vi "Save_SpectralGateSweep.vi"(0 "Refnum in":refnum<k34>, 1 "Integrated Emission":dbl[](array[numeric]), 2 "Capture number":i32, 7 "Image":dbl[][](array[numeric]), 11 "error in (no error)":errorcluster, 12 "Gate Delay array":dbl[](array[numeric]), 13 "Wavelength Array":dbl[](array[numeric])) -> (4 "Refnum out":refnum<k34>, 15 "error out":errorcluster)   [LabVIEW 2017]
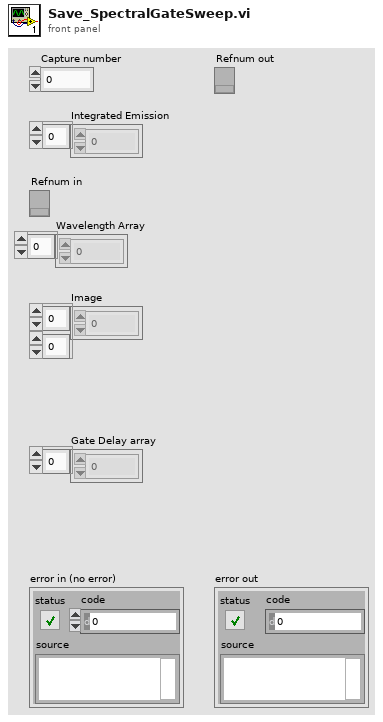
[diagram p1: front panel]
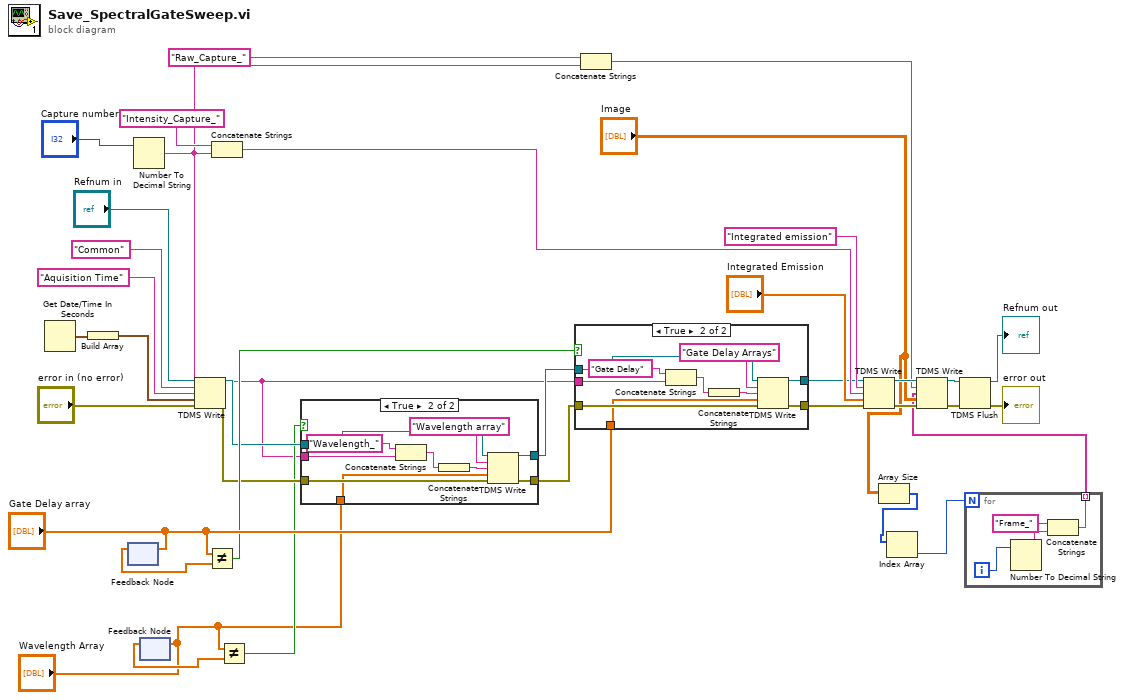
[diagram p0: block diagram]
diagram:
  n1 = Get Date/Time In Seconds() -> (seconds since 1Jan1904=w14:timestamp)
  n2 = Build Array(w14) -> (w19:timestamp[])
  n3 = feedback #1() -> (w17:dbl[])  [unwired: 1 in]
  n4 = feedback-in #1("Gate Delay array") -> ()
  n5 = Number To Decimal String(number="Capture number") -> (decimal integer string=w1:string)  [unwired: 1 in]
  n6 = feedback #2() -> (w4:dbl[])  [unwired: 1 in]
  n7 = feedback-in #2("Wavelength Array") -> ()
  n8 = TDMS Write(0:"Refnum in", 5:"Common" ("group name in (Untitled)"), 7:"Aquisition Time", 9:w19, 11:"error in (no error)") -> (4:w8:refnum<k34>, 15:w7:errorcluster)  [unwired: 1 in, 2 out]
  n9 = Not Equal?(x="Gate Delay array", y=w17) -> (x != y?=w15:bool)
  n10 = Concatenate Strings("Intensity_Capture_" ("group name in (Untitled)"), w1) -> (w24:string)
  n11 = Not Equal?(x="Wavelength Array", y=w4) -> (x != y?=w3:bool)
  n12 = case shown="True" w3 {
    tunnel: w8 -> [w38 w48]
    tunnel: w7 -> [w37 w47]
    tunnel: [w38 w46] -> w6
    tunnel: [w37 w45] -> w5
    tunnel: "Wavelength Array" -> [_ w42]
    tunnel: w1 -> [_ w39]
    frame False {
    }
    frame True {
      n13 = Concatenate Strings("Wavelength_" ("string"), w39) -> (w41:string)
      n14 = Concatenate Strings(w41) -> (w43:string)
      n15 = TDMS Write(0:w48, 5:"Wavelength array" ("group name in (Untitled)"), 7:w43, 9:w42, 11:w47) -> (4:w46:refnum<k34>, 15:w45:errorcluster)  [unwired: 1 in, 2 out]
    }
  }
  n16 = case shown="True" w15 {
    tunnel: w6 -> [w50 w60]
    tunnel: w5 -> [w49 w59]
    tunnel: [w50 w58] -> w21
    tunnel: [w49 w57] -> w22
    tunnel: "Gate Delay array" -> [_ w54]
    tunnel: w1 -> [_ w51]
    frame False {
    }
    frame True {
      n17 = Concatenate Strings("Gate Delay" ("string"), w51) -> (w53:string)
      n18 = Concatenate Strings(w53) -> (w55:string)
      n19 = TDMS Write(0:w60, 5:"Gate Delay Arrays" ("group name in (Untitled)"), 7:w55, 9:w54, 11:w59) -> (4:w58:refnum<k34>, 15:w57:errorcluster)  [unwired: 1 in, 2 out]
    }
  }
  n20 = Concatenate Strings("Raw_Capture_" ("group name in (Untitled)"), w1) -> (w28:string)
  n21 = TDMS Write(0:w21, 5:"Integrated emission" ("group name in (Untitled)"), 7:w24, 9:"Integrated Emission", 11:w22) -> (4:w29:refnum<k34>, 15:w30:errorcluster)  [unwired: 1 in, 2 out]
  n22 = Array Size(array="Image") -> (size(s)=w12:i32[])
  n23 = Index Array(array=w12) -> (element=w11:i32)  [unwired: 1 in]
  n24 = for {
    N: w11 -> [_]
    tunnel: [w61] -> w10 mode=indexing
    i -> [w64]
    n25 = Number To Decimal String(number=w64) -> (decimal integer string=w63:string)  [unwired: 1 in]
    n26 = Concatenate Strings("Frame_" ("string"), w63) -> (w61:string)
  }
  n27 = TDMS Write(0:w29, 5:w28, 7:w10, 9:"Image", 11:w30) -> (4:w25:refnum<k34>, 15:w26:errorcluster)  [unwired: 1 in, 2 out]
  n28 = TDMS Flush(4:w26, 7:w25) -> (0:→"error out":errorcluster, 3:→"Refnum out":refnum<k34>)
